vi "Launch Plot.vi"(8 "error in (no error)":errorcluster, 9 "Plot type":T1, 10 "File Path Control":path, 11 "Application Controller in":refnum<class "Application Controller.lvclass">) -> (0 "error out":errorcluster, 2 "Nested Actor's Enqueuer":refnum<class "Message Enqueuer.lvclass">, 3 "Application Controller out":refnum<class "Application Controller.lvclass">)   [LabVIEW 2016, in "Application Controller.lvclass"]
uses:
  Application Controller.lvclass
  Plots/Plot types.ctl
  <vilib>/ActorFramework/Message Enqueuer/Message Enqueuer.lvclass
  Plots/XY WFRM Plot/XY WFRM Plot.lvclass
  D:/github/Measure_core/Plots/Plot/Plot.lvclass
  Plots/XY WFRM Plot/XY WFRM Plot.lvclass/XY WFRM Plot.ctl
  Plots/XY Plot/XY Plot.lvclass
  Application Controller.lvclass/Application Controller.ctl
  Plots/Plot Messages/Add file Msg/Add file Msg.lvclass/Add file Msg.ctl
  <vilib>/ActorFramework/Message Enqueuer/Message Enqueuer.lvclass/Message Enqueuer.ctl
  Plots/XY WFRM Plot/Write Plot type.vi
  <vilib>/ActorFramework/Message Enqueuer/Enqueue.vi
  Plots/Plot/Plot.lvclass
  D:/github/Measure_core/Da Base/Da Base.lvclass
  Plots/Plot Messages/Add file Msg/Add file Msg.lvclass
  D:/Program Files/National Instruments/LabVIEW 2016/vi.lib/ActorFramework/Message/Message.lvclass
  Da Base Messages/Open Front Panel Msg/Open Front Panel Msg.lvclass
  <vilib>/ActorFramework/Message Priority Queue/Priority Enqueue.vi
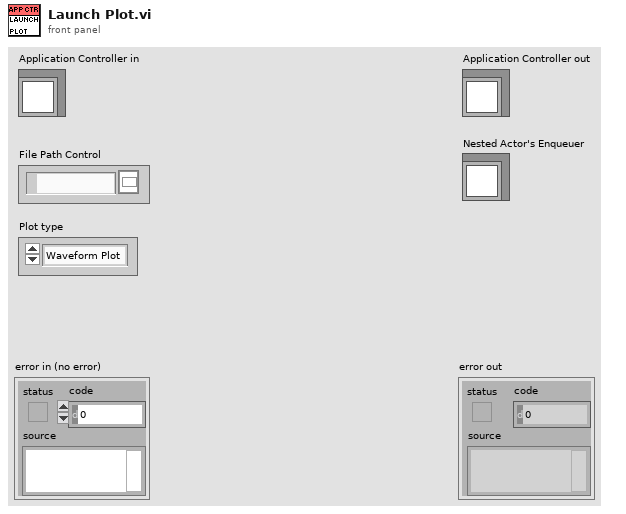
[diagram p1: front panel]
types:
  T1 = typedef "Plot types.ctl" = enum16{"Waveform Plot", "XY Plot", "Full XY"}
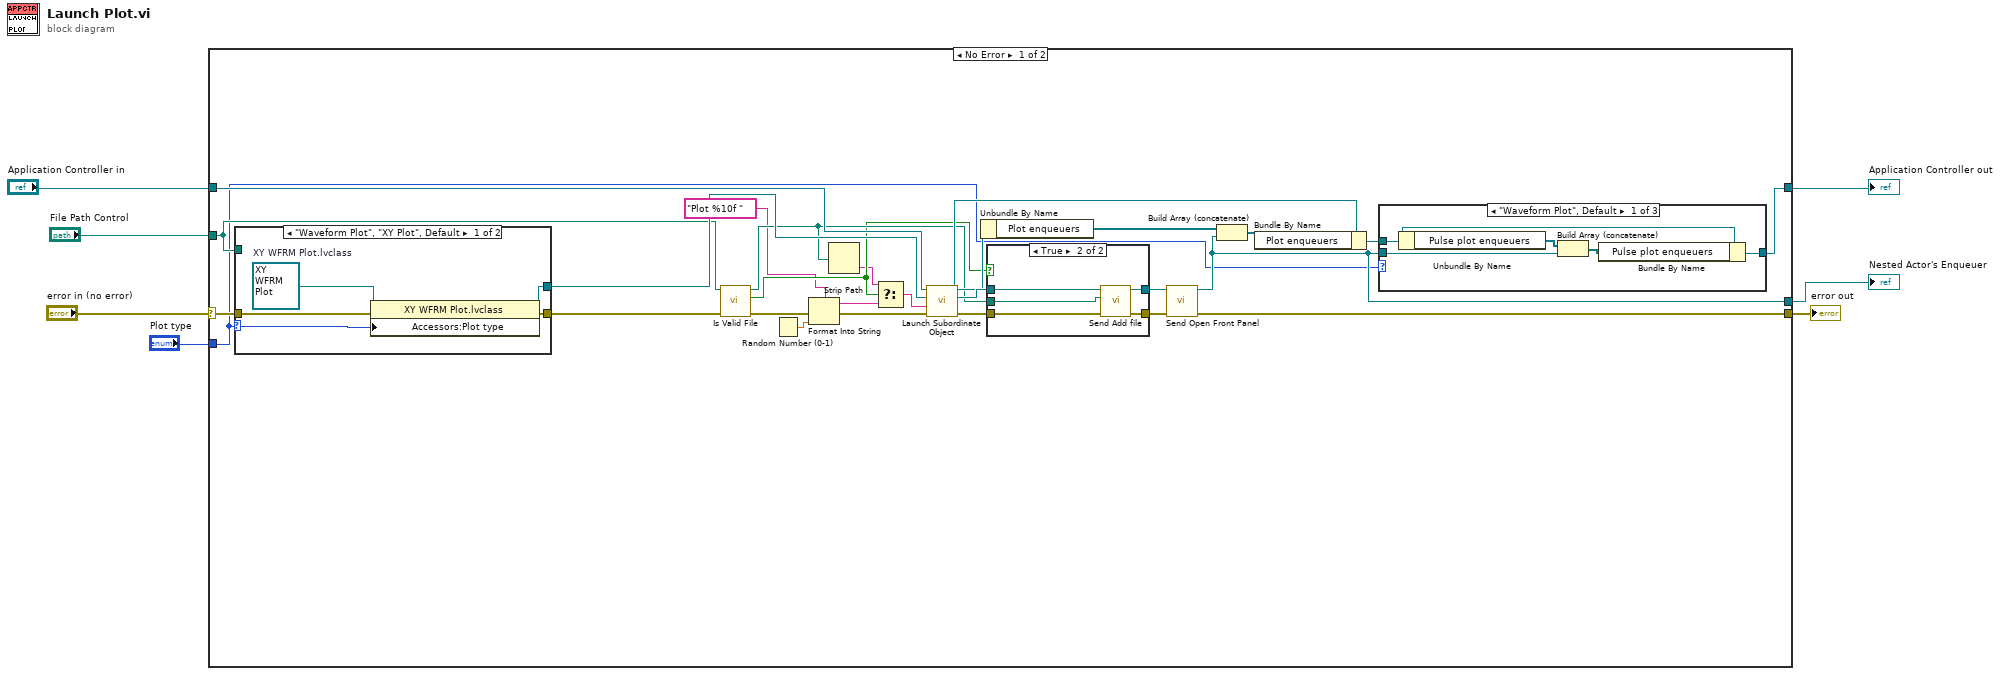
[diagram p0: block diagram]
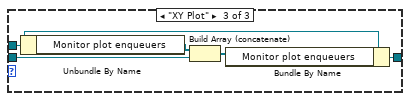
[diagram p3: hidden frame]
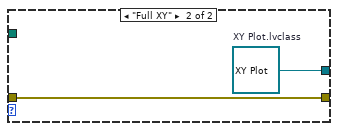
[diagram p5: hidden frame]
diagram:
  n1 = case shown="No Error" "error in (no error)" {
    selector: "error in (no error)" -> [w31 w60]
    tunnel: [w32 w60] -> w6
    tunnel: [w8 w59] -> w4
    tunnel: "Application Controller in" -> [w33 w59]
    tunnel: "File Path Control" -> [w23 _]
    tunnel: "Plot type" -> [w9 _]
    tunnel: [w10 _] -> w1
    frame No Error {
      n2 = case shown="\"Waveform Plot\", \"XY Plot\", Default" w9 {
        selector: w9 -> [w52 _]
        tunnel: [w54 w58] -> w30
        tunnel: w23 -> [_ _]
        tunnel: [w53 w57] -> w22
        tunnel: w31 -> [w55 w57]
        frame "Waveform Plot", "XY Plot", Default {
          w56 = refnum<class "XY WFRM Plot.lvclass"> refnum  # XY WFRM Plot.lvclass
          n3 = property class="XY WFRM Plot.lvclass"(reference=w56, error in=w55, "Accessors:Plot type"=w52) -> (reference out=w54:refnum<class "XY WFRM Plot.lvclass">, error out=w53:errorcluster)
        }
        frame "Full XY" {
          w58 = refnum<class "XY Plot.lvclass"> refnum  # XY Plot.lvclass
        }
      }
      n4 = call "Is Valid File.vi"("Error In"=w22, "File"=w23) -> ("Error Out"=w12:errorcluster, "Valid file"=w19:bool, "File out"=w20:path)  [unwired: 7 in]
      n5 = Random Number (0-1)() -> (number: 0 to 1=w17:dbl)
      n6 = Format Into String(format string="Plot %10f ", error in=w12, w17) -> (resulting string=w15:string, error out=w13:errorcluster)  [unwired: 1 in]
      n7 = Strip Path(path=w20) -> (name=w18:string)  [unwired: 1 out]
      n8 = Select(t=w18, s=w19, f=w15) -> (s? t:f=w14:string)
      n9 = call-dynamic "Launch Subordinate Object.vi"("error in (no error)"=w13, "Name"=w14, "Subordinate Object"=w30, "Measure Object in"=w33) -> ("error out"=w21:errorcluster, "Nested Actor's Enqueuer"=w29:refnum<class "Message Enqueuer.lvclass">, "Measure Object out"=w26:refnum<class "Application Controller.lvclass">)  [unwired: 5 in]
      n10 = Unbundle By Name(w26) -> ("Plot enqueuers"=w25:refnum<class "Message Enqueuer.lvclass">[])
      n11 = case shown="True" w19 {
        tunnel: w29 -> [w46 w51]
        tunnel: [w46 w50] -> w28
        tunnel: [w45 w49] -> w27
        tunnel: w21 -> [w45 w48]
        tunnel: w20 -> [_ w47]
        frame False {
        }
        frame True {
          n12 = call "Send Add file.vi"("error in (no error)"=w48, "File Path Control"=w47, "Message Enqueuer"=w51) -> ("error out"=w49:errorcluster, "Message Enqueuer out"=w50:refnum<class "Message Enqueuer.lvclass">)  [unwired: 7 in]
        }
      }
      n13 = call "Send Open Front Panel.vi"("error in (no error)"=w27, "Message Enqueuer"=w28) -> ("error out"=w32:errorcluster, "Message Enqueuer out"=w10:refnum<class "Message Enqueuer.lvclass">)  [unwired: 8 in]
      n14 = Build Array (concatenate)(w25, w10) -> (w24:refnum<class "Message Enqueuer.lvclass">[])
      n15 = Bundle By Name(cluster=w26, "Plot enqueuers"=w24) -> (w11:refnum<class "Application Controller.lvclass">)
      n16 = case shown="\"Waveform Plot\", Default" w9 {
        tunnel: w11 -> [w36 w39 w42]
        tunnel: w10 -> [w37 _ w43]
        tunnel: [w34 w39 w40] -> w8
        frame "Waveform Plot", Default {
          n17 = Unbundle By Name(w36) -> ("Pulse plot enqueuers"=w38:refnum<class "Message Enqueuer.lvclass">[])
          n18 = Build Array (concatenate)(w38, w37) -> (w35:refnum<class "Message Enqueuer.lvclass">[])
          n19 = Bundle By Name(cluster=w36, "Pulse plot enqueuers"=w35) -> (w34:refnum<class "Application Controller.lvclass">)
        }
        frame "Full XY" {
        }
        frame "XY Plot" {
          n20 = Unbundle By Name(w42) -> ("Monitor plot enqueuers"=w44:refnum<class "Message Enqueuer.lvclass">[])
          n21 = Build Array (concatenate)(w44, w43) -> (w41:refnum<class "Message Enqueuer.lvclass">[])
          n22 = Bundle By Name(cluster=w42, "Monitor plot enqueuers"=w41) -> (w40:refnum<class "Application Controller.lvclass">)
        }
      }
    }
    frame Error {
    }
  }
  "error out" <- w6
  "Application Controller out" <- w4
  "Nested Actor's Enqueuer" <- w1
